vi "svx_Get DAQmx Info.vi"(0 "task in":refnum<k21>, 5 "active channels":refnum<k21>, 7 "AI channel settings":T1={"max value [V]"=10.0, "min value [V]"=10.0, "terminal config"=10083, "DSA channel settings"={"coupling"=10045, "enable IEPE excitation"=FALSE, "IEPE current [mA]"=4.0}} {"DSA channel settings"."IEPE current [mA]" min=0.0 max=20.0 format="%.1f"; "DSA channel settings"."coupling" items=["AC"=10045, "DC"=10050, "GND"=10066]; "min value [V]" format="%.2f"; "terminal config" items=["Default"=-1, "RSE"=10083, "NRSE"=10078, "Differential"=10106, "Pseudodifferential"=12529]; "max value [V]" format="%.2f"}, 11 "error in (no error)":errorcluster) -> (4 "task out":refnum<k21>, 15 "error out":errorcluster)   [LabVIEW 2017]
uses:
  <vilib>/addons/_NISVFA/_Shared subVIs/Controls/svc_Channel Settings.ctl
  <vilib>/addons/_NISVFA/_Shared subVIs/Controls/svc_DSA Channel Settings.ctl
  <resource>/objmgr/daqmx.rc
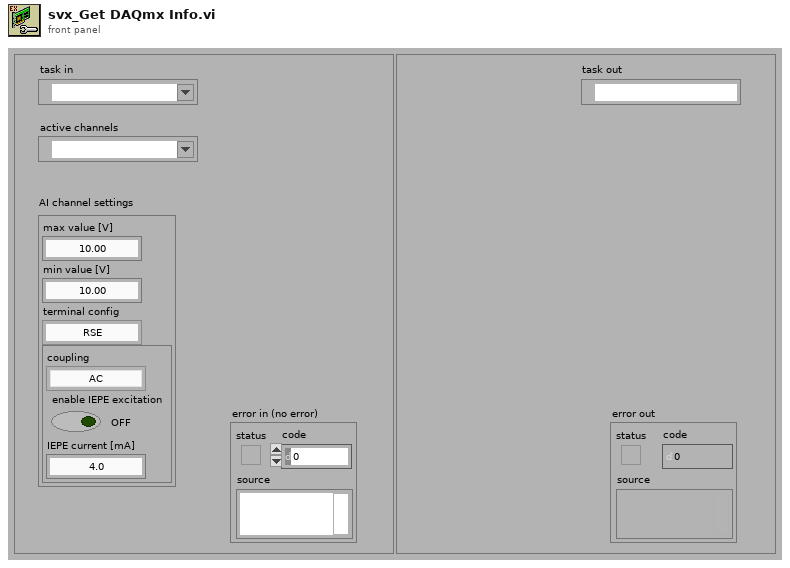
[diagram p1: front panel]
types:
  T1 = typedef "svc_Channel Settings.ctl" = cluster{"max value [V]":dbl, "min value [V]":dbl, "terminal config":i32, "DSA channel settings":T2}
  T2 = typedef "svc_DSA Channel Settings.ctl" = cluster{"coupling":i32, "enable IEPE excitation":bool, "IEPE current [mA]":dbl}
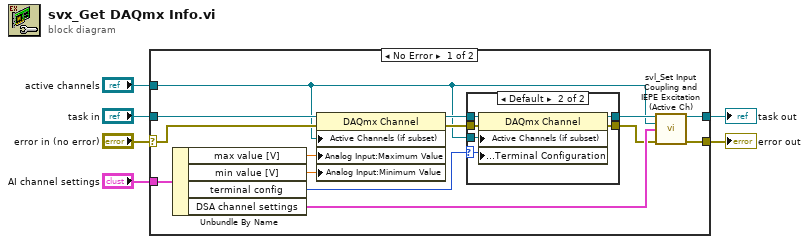
[diagram p0: block diagram]
diagram:
  n1 = case shown="No Error" "error in (no error)" {
    selector: "error in (no error)" -> [w13 w29]
    tunnel: "AI channel settings" -> [w17 _]
    tunnel: [w15 w30] -> w6
    tunnel: "task in" -> [w18 w30]
    tunnel: [w14 w29] -> w3
    tunnel: "active channels" -> [w7 _]
    frame No Error {
      n2 = Unbundle By Name(w17) -> ("max value [V]"=w20:dbl, "min value [V]"=w19:dbl, "terminal config"=w8:i32, "DSA channel settings"=w16:T2)
      n3 = property class="DAQmx Channel"(reference=w18, error in=w13, "Active Channels (if subset)"=w7, "Analog Input:Maximum Value"=w20, "Analog Input:Minimum Value"=w19) -> (reference out=w12:refnum<k21>, error out=w11:errorcluster)
      n4 = case shown="Default" w8 {
        selector: w8 -> [_ w24]
        tunnel: w12 -> [w22 w28]
        tunnel: w11 -> [w21 w27]
        tunnel: [w21 w26] -> w10
        tunnel: [w22 w25] -> w9
        tunnel: w7 -> [_ w23]
        frame -1 {
        }
        frame Default {
          n5 = property class="DAQmx Channel"(reference=w28, error in=w27, "Active Channels (if subset)"=w23, "Analog Input:General Properties:Input Configuration:Terminal Configuration"=w24) -> (reference out=w25:refnum<k21>, error out=w26:errorcluster)
        }
      }
      n6 = call <vilib>:"svl_Set Input Coupling and IEPE Excitation (Active Ch).vi"("AI task name"=w9, "active channels"=w7, "DSA channel settings"=w16, "error in (no error)"=w10) -> ("dup AI task name"=w15:refnum<k21>, "error out"=w14:errorcluster)  [unwired: 10 in]
    }
    frame Error {
    }
  }
  "error out" <- w3
  "task out" <- w6
